vi "Set Event-Timer.vi"(8 "error in (no error)":errorcluster, 10 "Event-Timer":u16, 11 "PDO Communication Parameter in":refnum<class "PDO Communication Parameter.lvclass">) -> (0 "error out":errorcluster, 3 "PDO Communication Parameter out":refnum<class "PDO Communication Parameter.lvclass">)   [LabVIEW 2020, in "CANopen.lvlib" / "PDO Communication Parameter.lvclass"]
uses:
  PDO Communication Parameter.lvclass
  PDO Communication Parameter.lvclass/PDO Communication Parameter.ctl
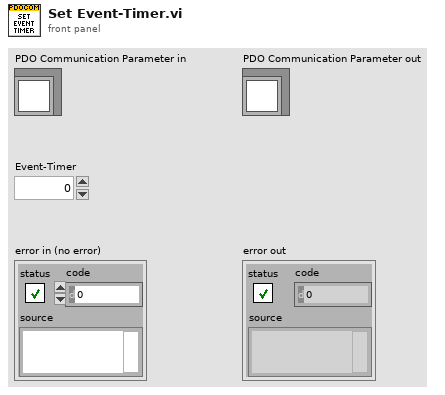
[diagram p1: front panel]
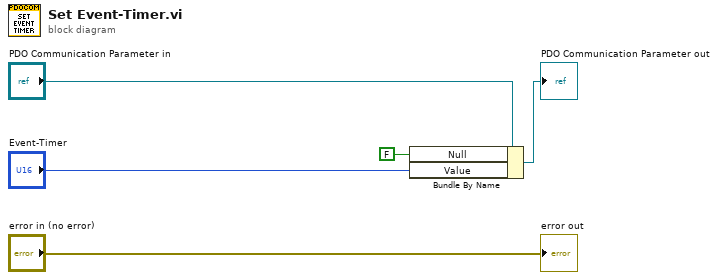
[diagram p0: block diagram]
diagram:
  n1 = Bundle By Name(cluster="PDO Communication Parameter in", "Null"=FALSE ("Event-Timer.Null"), "Value"="Event-Timer") -> (→"PDO Communication Parameter out":refnum<class "PDO Communication Parameter.lvclass">)
  "error out" <- "error in (no error)"
